vi "Get Test Running State.vi"(8 "error in (no error)":errorcluster) -> (0 "error out":errorcluster, 2 "Last Test Start Time":timestamp, 3 "Is Test Running":bool)   [LabVIEW 2020, in "FlexLoggerTagHelpers.lvlib"]
uses:
  FlexLoggerTagHelpers.lvlib
  <vilib>/Skyline/Tag/Shared/typedefs/DataType.ctl
  System Tags.ctl
  <vilib>/Skyline/Tag/Wrapper/Wrapper AMQP_class/Open Tag AMQP.vi
  <vilib>/Skyline/Tag/Wrapper/Wrapper_class/Read Tag (Timestamp).vi
  <vilib>/Skyline/Tag/Wrapper/Wrapper_class/Close Tag (Single).vi
  <vilib>/Skyline/Tag/Wrapper/Wrapper_class/Read Tag (Boolean).vi
  <vilib>/Skyline/Tag/Wrapper/Wrapper_class/NI Skyline Tag.lvclass
  <vilib>/Skyline/Tag/Wrapper/Wrapper AMQP_class/NI Skyline Tag AMQP.lvclass
  <vilib>/Skyline/Tag/Shared/NI Skyline Tag.lvlib
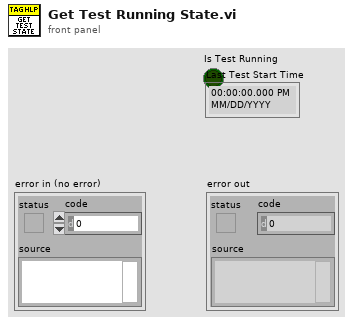
[diagram p1: front panel]
types:
  T1 = typedef "FlexLoggerTagHelpers.lvlib/System Tags.ctl" = enum16{"LastTestStart", "IsTestSessionRunning"}
  T2 = typedef "NI Skyline Tag.lvlib/DataType.ctl" = enum32{"Double", "I32", "String", "Boolean", "U64", "Timestamp"}
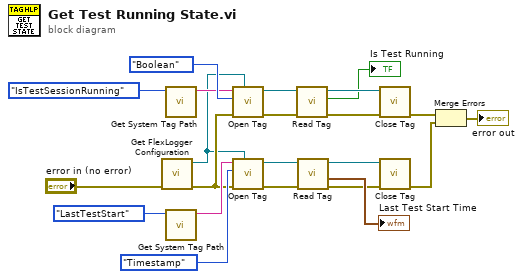
[diagram p0: block diagram]
diagram:
  n1 = call "Get FlexLogger Configuration.vi"("error in (no error)"="error in (no error)") -> ("error out"=w3:errorcluster, "Local FlexLogger Configuration"=w1:refnum<class "NI Skyline Configuration AMQP.lvclass">)  [unwired: 9 in]
  n2 = call "Get System Tag Path.vi"("sytem tag"=System_Tags."IsTestSessionRunning") -> ("tag path"=w17:string)  [unwired: 10 in]
  n3 = call "Get System Tag Path.vi"("sytem tag"=System_Tags."LastTestStart" ("SystemTag")) -> ("tag path"=w18:string)  [unwired: 10 in]
  n4 = call-poly <vilib>:"Open Tag.vi"("configuration"=w1, "error in (no error)"=w3, "data type"=DataType."Boolean", "path"=w17) -> ("error out"=w13:errorcluster, "tag"=w16:refnum<class "NI Skyline Tag.lvclass">)  [unwired: 6 in]
  n5 = call-poly <vilib>:"Open Tag.vi"("configuration"=w1, "error in (no error)"=w3, "data type"=DataType."Timestamp", "path"=w18) -> ("error out"=w12:errorcluster, "tag"=w20:refnum<class "NI Skyline Tag.lvclass">)  [unwired: 6 in]
  n6 = call-poly <vilib>:"Read Tag.vi"("error in (no error)"=w13, "tag in"=w16) -> ("error out"=w9:errorcluster, "value"=→"Is Test Running":bool, "tag out"=w10:refnum<class "NI Skyline Tag.lvclass">)  [unwired: 5 in, 2 out]
  n7 = call-poly <vilib>:"Read Tag.vi"("error in (no error)"=w12, "tag in"=w20) -> ("error out"=w11:errorcluster, "time stamp"=→"Last Test Start Time":timestamp, "tag out"=w14:refnum<class "NI Skyline Tag.lvclass">)  [unwired: 5 in, 2 out]
  n8 = call-poly <vilib>:"Close Tag.vi"("error in (no error)"=w9, "tag"=w10) -> ("error out"=w8:errorcluster)  [unwired: 9 in]
  n9 = call-poly <vilib>:"Close Tag.vi"("error in (no error)"=w11, "tag"=w14) -> ("error out"=w7:errorcluster)  [unwired: 9 in]
  n10 = Merge Errors(w8, w7) -> (→"error out":errorcluster)
